vi "enum wrap 2.vi"() -> ()   [LabVIEW 2013]
panel:
  out "x+y":u16
  in  "stop":bool
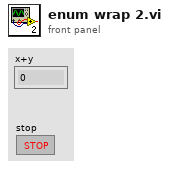
[diagram p1: front panel]
types:
  T1 = enum16{"", "1", "2", "3", "4", "5", "6", "7", "8", "9", "10", "11", "12", "13", "14"}
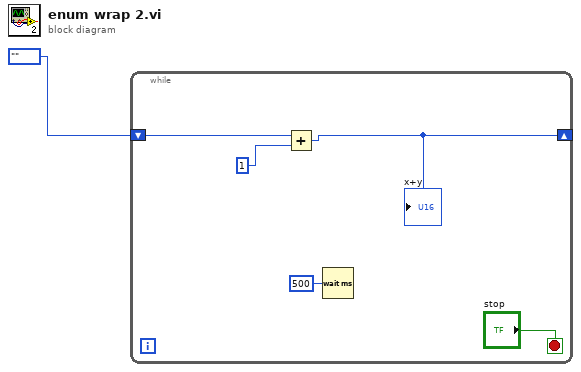
[diagram p0: block diagram]
diagram:
  n1 = while {
    shift-right: [w4] -> _
    shift-left: T1."" -> [w6]
    stop <- "stop" stop-if-true
    n2 = Add(x=w6, y=1) -> (x+y=w4:i32)
    "x+y" <- w4
    n3 = Wait (ms)(milliseconds to wait=u32 500) -> ()  [unwired: 1 out]
  }
